vi "Write On Off Status.vi"(8 "error in (no error)":errorcluster, 10 "On Off Status":dbl format="%#_13g", 11 "ThermotronDriver in":refnum<class "ThermotronDriver.lvclass">) -> (0 "error out":errorcluster, 3 "ThermotronDriver out":refnum<class "ThermotronDriver.lvclass">)   [LabVIEW 2023, in "ThermotronDriver.lvlib" / "ThermotronDriver.lvclass"]
uses:
  ThermotronDriver.lvclass
  ThermotronDriver.lvclass/ThermotronDriver.ctl
  <vilib>/ADAS Replay HIL/Channels/Tag Wrapper/Tag Wrapper.lvlib
  <vilib>/ADAS Replay HIL/Channels/Tag Wrapper/Polymorphic/Write Channel (Double).vi
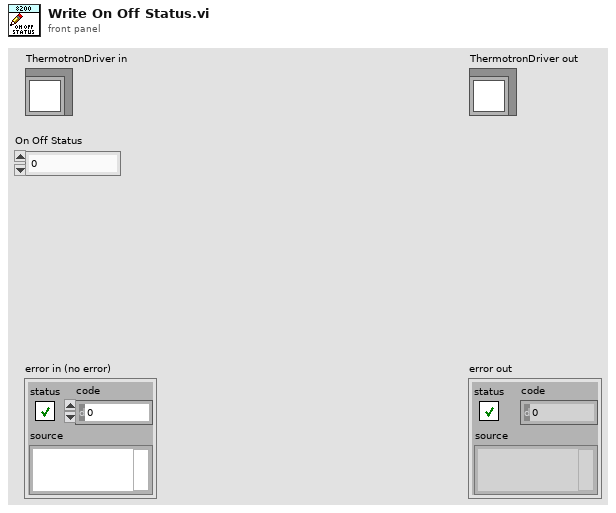
[diagram p1: front panel]
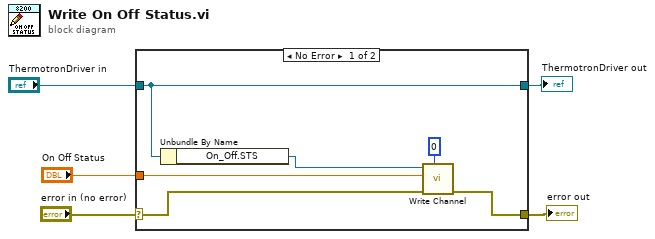
[diagram p0: block diagram]
diagram:
  n1 = case shown="No Error" "error in (no error)" {
    selector: "error in (no error)" -> [w10 w13]
    tunnel: [w9 w13] -> w4
    tunnel: [w11 w12] -> w2
    tunnel: "ThermotronDriver in" -> [w11 w12]
    tunnel: "On Off Status" -> [w6 _]
    frame No Error {
      n2 = Unbundle By Name(w11) -> ("On_Off.STS"=w8:refnum<k21>)
      n3 = call-poly <vilib>:"Write Channel.vi"("Timeout (ms)"=0, "error in"=w10, "Value to Write"=w6, "ADAS HIL Channel in"=w8) -> ("error out"=w9:errorcluster)  [unwired: 5 in, 2 out]
    }
    frame Error {
    }
  }
  "error out" <- w4
  "ThermotronDriver out" <- w2
